vi "setUp.vi"(8 "error in (no error)":errorcluster, 11 "reference in":refnum<class "Verify IMemento.lvclass">) -> (0 "error out":errorcluster, 3 "reference in":refnum<class "Verify IMemento.lvclass">)   [LabVIEW 2009, in "Verify IMemento.lvclass"]
doc: "setUp runs prior to the test method during test execution. Use this method to initialize any object data required by your tests."
uses:
  Verify IMemento.lvclass
  Verify IMemento.lvclass/Verify IMemento.ctl
  <vilib>/addons/_JKI Toolkits/VI Tester/TestCase.llb/TestCase.lvclass
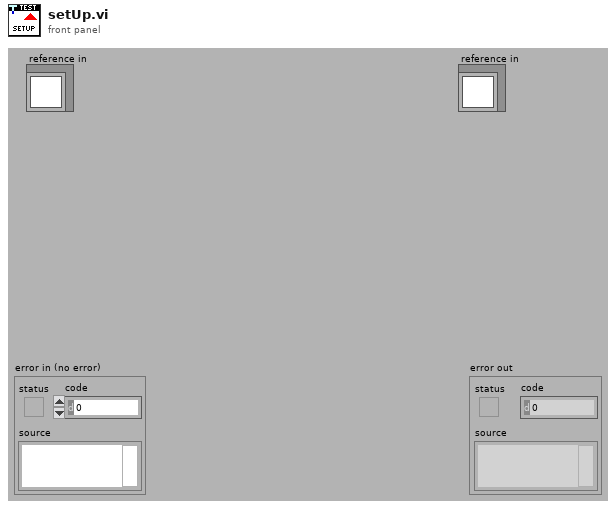
[diagram p1: front panel]
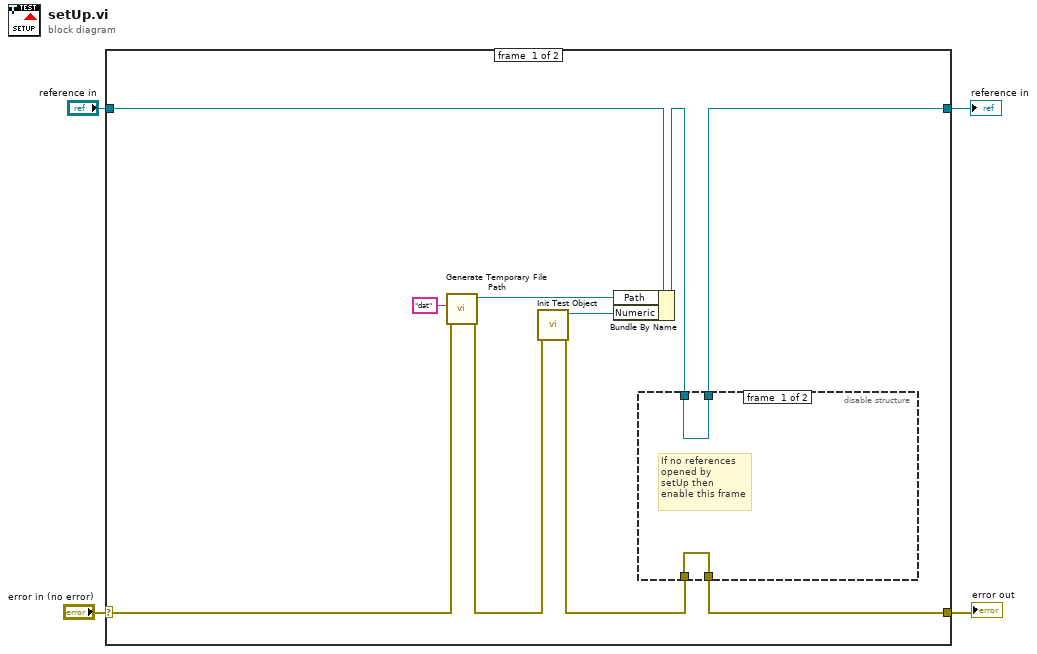
[diagram p0: block diagram]
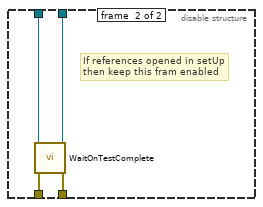
[diagram p2: hidden frame]
diagram:
  n1 = case shown="No Error" "error in (no error)" {
    selector: "error in (no error)" -> [w6 w22]
    tunnel: [w11 w22] -> w3
    tunnel: [w12 w21] -> w1
    tunnel: "reference in" -> [w14 w21]
    frame #0 {
      n2 = call <vilib>:"Generate Temporary File Path.vi"("error in (no error)"=w6, "Temporary File Extension (tmp)"="dat") -> ("error out"=w5:errorcluster, "Unique Temporary File Path"=w8:path)  [unwired: 8 in]
      n3 = call "Init Test Object.vi"("error in (no error)"=w5) -> ("error out"=w9:errorcluster, "Numeric out"=w10:refnum<class "Numeric Test Object.lvclass">)  [unwired: 9 in]
      n4 = Bundle By Name(cluster=w14, "Path"=w8, "Numeric"=w10) -> (w13:refnum<class "Verify IMemento.lvclass">)
      n5 = disable-structure shown="Enabled" {
        disable-tunnel: w13 -> [w16 w20]
        disable-tunnel: [w16 w19] -> w12
        disable-tunnel: w9 -> [w15 w18]
        disable-tunnel: [w15 w17] -> w11
        frame #0 {
          # "If no references opened by\nsetUp then enable this frame"
        }
        frame #1 {
          # "If references opened in setUp\nthen keep this fram enabled"
          n6 = call <vilib>:"WaitOnTestComplete.vi"("error in (no error)"=w18, "TestCase in"=w20) -> ("error out"=w17:errorcluster, "TestCase out"=w19:refnum<class "Verify IMemento.lvclass">)  [unwired: 8 in]
        }
      }
    }
    frame #1 {
    }
  }
  "error out" <- w3
  "reference in" <- w1
